vi "Update Started Tree Symbol.vi"(8 "error in":errorcluster, 10 "test GUID":string, 11 "Test Hierarchy Tree":refnum<vi>) -> ()   [LabVIEW 2011, in "GraphicalTestRunner.lvlib"]
uses:
  GraphicalTestRunner.lvlib
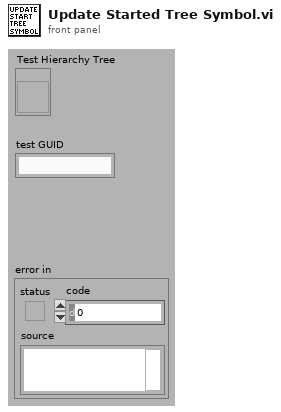
[diagram p1: front panel]
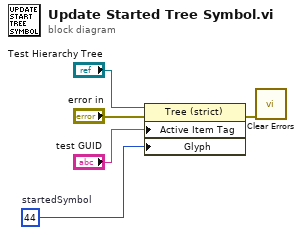
[diagram p0: block diagram]
diagram:
  w2 = 44  # startedSymbol
  n1 = property class="Tree (strict)"(reference="Test Hierarchy Tree", error in="error in", "Active Item Tag"="test GUID", "Glyph"=w2) -> (error out=w5:errorcluster)  [unwired: 1 out]
  n2 = call <vilib>:"Clear Errors.vi"("error in (no error)"=w5) -> ()  [unwired: 6 in, 1 out]
